vi "RandBigPrime.vi"(1 "Numeric":i16) -> (0 "Random Prime (1e18)":cluster{"Boolean":bool, "Array":u64[]})   [LabVIEW 2023]
panel:
  out "Is Prime 4":bool
  out "Is Prime 3":bool
  out "Is Prime 2":bool
  out "Is Prime":bool
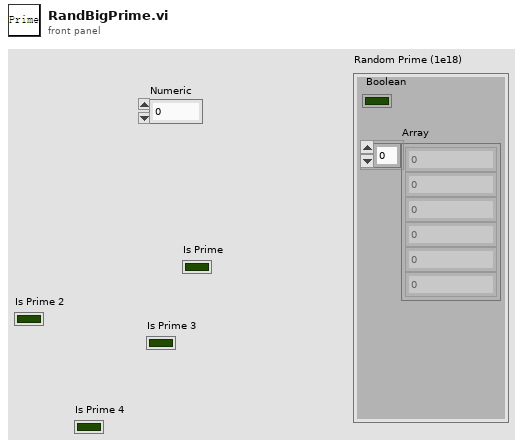
[diagram p1: front panel]
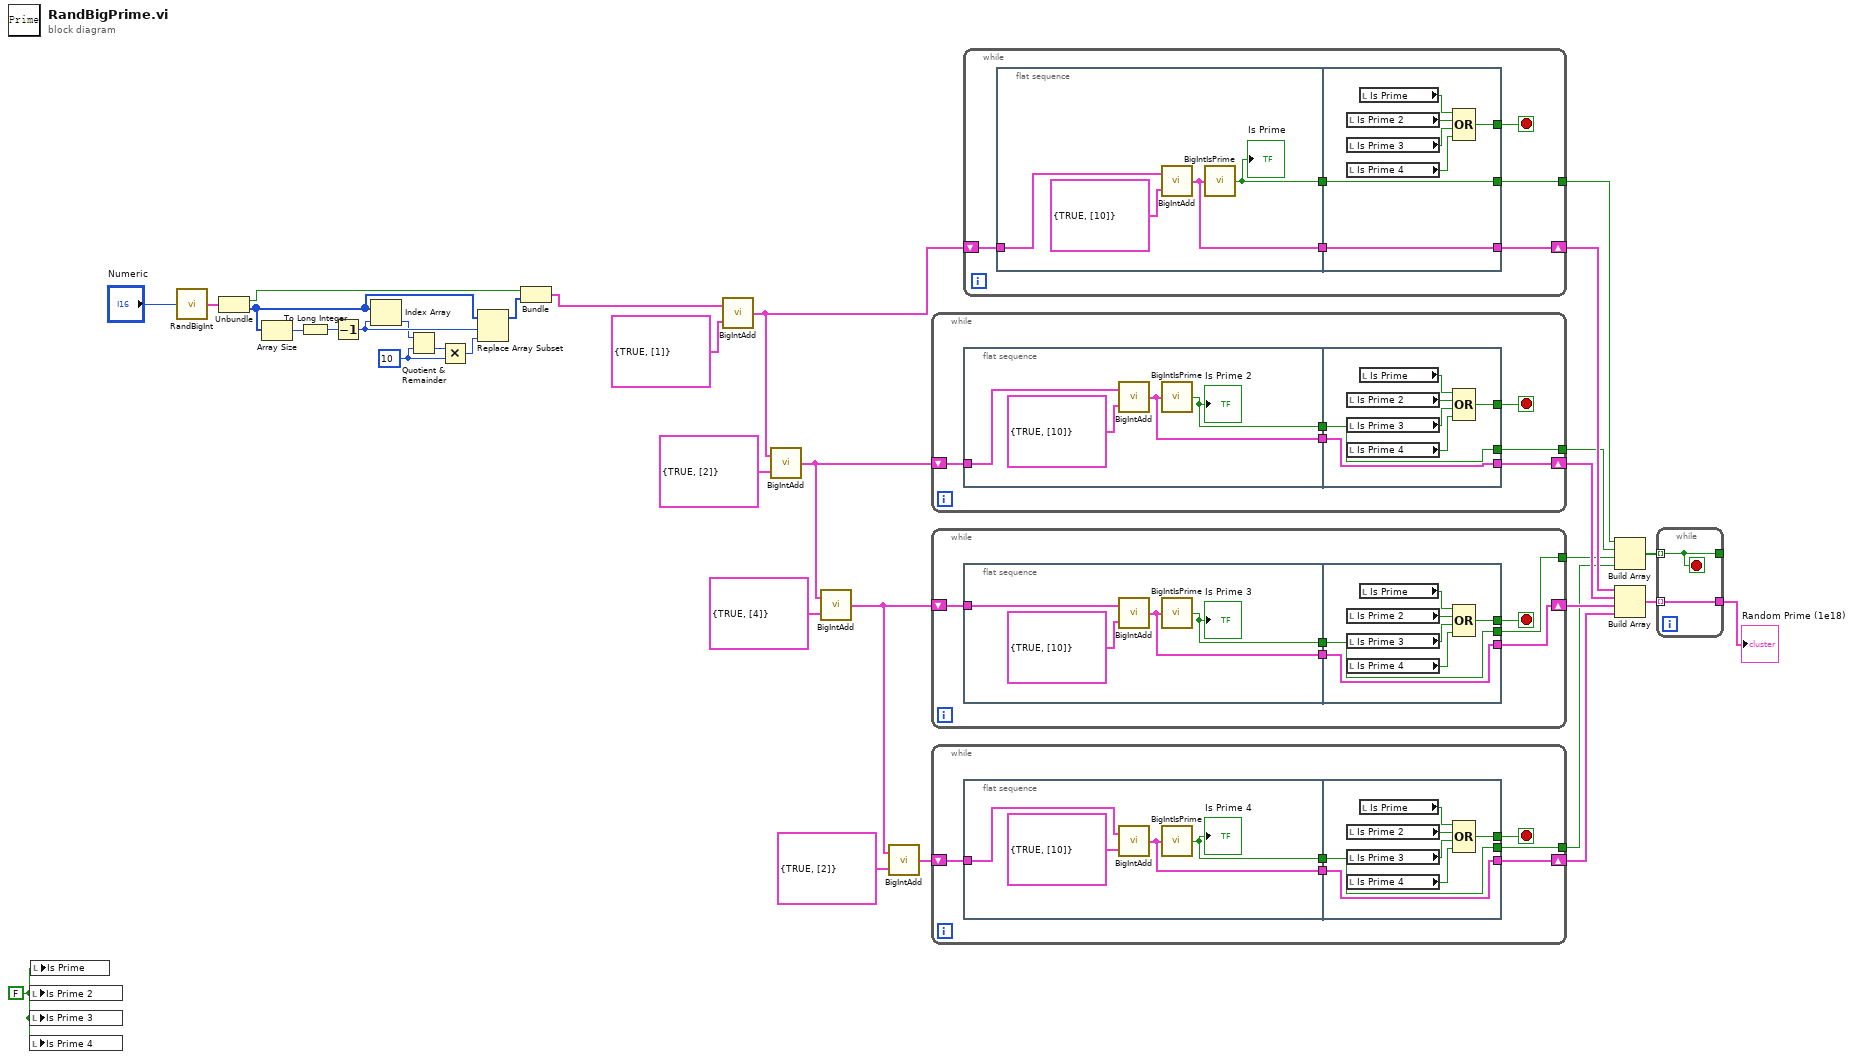
[diagram p0: block diagram]
diagram:
  w5 = u64 10
  w8 = FALSE
  n1 = local write "Is Prime 2"(w8) -> ()
  n2 = local write "Is Prime 3"(w8) -> ()
  n3 = local write "Is Prime 4"(w8) -> ()
  n4 = local write "Is Prime"(w8) -> ()
  n5 = call "RandBigInt.vi"("length (x1e9)"="Numeric") -> ("Random Number"=w33:cluster{"P/N":bool, "Array":u64[]})
  n6 = Unbundle(w33) -> ("P/N"=w30:bool, "Array"=w2:u64[])
  n7 = Array Size(array=w2) -> (size(s)=w1:i32)
  n8 = To Long Integer(number=w1) -> (32bit integer=w29:i32)
  n9 = Decrement(x=w29) -> (x-1=w32:i32)
  n10 = Index Array(array=w2, index=w32) -> (element=w7:u64)
  n11 = Quotient & Remainder(x=w7, y=w5) -> (floor(x/y)=w6:u64)  [unwired: 1 out]
  n12 = Multiply(x=w6, y=w5) -> (x*y=w4:u64)
  n13 = Replace Array Subset(array=w2, new element=w4, index=w32) -> (w31:u64[])
  n14 = Bundle("P/N"=w30, "Array"=w31) -> (w9:cluster{"P/N":bool, "Array":u64[]})  [unwired: 1 in]
  n15 = call "BigIntAdd.vi"("b"=cluster{bool, u64[]} {TRUE, [1]}, "a"=w9) -> ("a + b"=w10:cluster{"Boolean":bool, "Array":u64[]})
  n16 = call "BigIntAdd.vi"("b"=cluster{bool, u64[]} {TRUE, [2]}, "a"=w10) -> ("a + b"=w24:cluster{"Boolean":bool, "Array":u64[]})
  n17 = call "BigIntAdd.vi"("b"=cluster{bool, u64[]} {TRUE, [4]}, "a"=w24) -> ("a + b"=w25:cluster{"Boolean":bool, "Array":u64[]})
  n18 = call "BigIntAdd.vi"("b"=cluster{bool, u64[]} {TRUE, [2]}, "a"=w25) -> ("a + b"=w23:cluster{"Boolean":bool, "Array":u64[]})
  n19 = while {
    shift-right: [w38] -> w21
    shift-left: w24 -> [w39]
    tunnel: [w37] -> w17
    stop <- w34 stop-if-true
    n20 = flat-sequence {
      tunnel: w39 -> [w43]
      tunnel: [w41] -> w36
      tunnel: [w40] -> w35
      tunnel: [w49] -> w37
      tunnel: [w50] -> w38
      tunnel: w36 -> [w50]
      tunnel: w35 -> [w49]
      tunnel: [w44] -> w34
      frame #0 {
        n21 = call "BigIntAdd.vi"("b"=cluster{bool, u64[]} {TRUE, [10]}, "a"=w43) -> ("a + b"=w41:cluster{"Boolean":bool, "Array":u64[]})
        n22 = call "BigIntIsPrime.vi"("a"=w41) -> ("Is Prime"=w40:bool)
        "Is Prime 2" <- w40
      }
      frame #1 {
        n23 = local read "Is Prime 2"() -> (w46:bool)
        n24 = local read "Is Prime 3"() -> (w47:bool)
        n25 = local read "Is Prime 4"() -> (w48:bool)
        n26 = local read "Is Prime"() -> (w45:bool)
        n27 = Compound Arithmetic op=OR(w45, w46, w47, w48) -> (w44:bool)
      }
    }
  }
  n28 = while {
    shift-right: [w55] -> w20
    shift-left: w25 -> [w56]
    tunnel: [w54] -> w16
    stop <- w51 stop-if-true
    n29 = flat-sequence {
      tunnel: w56 -> [w60]
      tunnel: [w58] -> w53
      tunnel: [w57] -> w52
      tunnel: [w66] -> w54
      tunnel: [w67] -> w55
      tunnel: w53 -> [w67]
      tunnel: w52 -> [w66]
      tunnel: [w61] -> w51
      frame #0 {
        n30 = call "BigIntAdd.vi"("b"=cluster{bool, u64[]} {TRUE, [10]}, "a"=w60) -> ("a + b"=w58:cluster{"Boolean":bool, "Array":u64[]})
        n31 = call "BigIntIsPrime.vi"("a"=w58) -> ("Is Prime"=w57:bool)
        "Is Prime 3" <- w57
      }
      frame #1 {
        n32 = local read "Is Prime 2"() -> (w63:bool)
        n33 = local read "Is Prime 3"() -> (w64:bool)
        n34 = local read "Is Prime 4"() -> (w65:bool)
        n35 = local read "Is Prime"() -> (w62:bool)
        n36 = Compound Arithmetic op=OR(w62, w63, w64, w65) -> (w61:bool)
      }
    }
  }
  n37 = while {
    shift-right: [w72] -> w19
    shift-left: w23 -> [w73]
    tunnel: [w71] -> w15
    stop <- w68 stop-if-true
    n38 = flat-sequence {
      tunnel: w73 -> [w77]
      tunnel: [w75] -> w70
      tunnel: [w74] -> w69
      tunnel: [w83] -> w71
      tunnel: [w84] -> w72
      tunnel: w70 -> [w84]
      tunnel: w69 -> [w83]
      tunnel: [w78] -> w68
      frame #0 {
        n39 = call "BigIntAdd.vi"("b"=cluster{bool, u64[]} {TRUE, [10]}, "a"=w77) -> ("a + b"=w75:cluster{"Boolean":bool, "Array":u64[]})
        n40 = call "BigIntIsPrime.vi"("a"=w75) -> ("Is Prime"=w74:bool)
        "Is Prime 4" <- w74
      }
      frame #1 {
        n41 = local read "Is Prime 2"() -> (w80:bool)
        n42 = local read "Is Prime 3"() -> (w81:bool)
        n43 = local read "Is Prime 4"() -> (w82:bool)
        n44 = local read "Is Prime"() -> (w79:bool)
        n45 = Compound Arithmetic op=OR(w79, w80, w81, w82) -> (w78:bool)
      }
    }
  }
  n46 = while {
    shift-right: [w89] -> w22
    shift-left: w10 -> [w90]
    tunnel: [w88] -> w18
    stop <- w85 stop-if-true
    n47 = flat-sequence {
      tunnel: w90 -> [w94]
      tunnel: [w92] -> w87
      tunnel: [w91] -> w86
      tunnel: [w100] -> w88
      tunnel: [w101] -> w89
      tunnel: w87 -> [w101]
      tunnel: w86 -> [w100]
      tunnel: [w95] -> w85
      frame #0 {
        n48 = call "BigIntAdd.vi"("b"=cluster{bool, u64[]} {TRUE, [10]}, "a"=w94) -> ("a + b"=w92:cluster{"Boolean":bool, "Array":u64[]})
        n49 = call "BigIntIsPrime.vi"("a"=w92) -> ("Is Prime"=w91:bool)
        "Is Prime" <- w91
      }
      frame #1 {
        n50 = local read "Is Prime 2"() -> (w98:bool)
        n51 = local read "Is Prime 3"() -> (w97:bool)
        n52 = local read "Is Prime 4"() -> (w96:bool)
        n53 = local read "Is Prime"() -> (w99:bool)
        n54 = Compound Arithmetic op=OR(w99, w98, w97, w96) -> (w95:bool)
      }
    }
  }
  n55 = Build Array(w18, w17, w16, w15) -> (w13:bool[])
  n56 = Build Array(w22, w21, w20, w19) -> (w14:cluster{"Boolean":bool, "Array":u64[]}[])
  n57 = while {
    tunnel: w14 -> [w103] mode=indexing
    tunnel: w13 -> [w102] mode=indexing
    tunnel: [w103] -> w12
    tunnel: [w102] -> _
    stop <- w102 stop-if-true
  }
  "Random Prime (1e18)" <- w12
